vi "TickInd (SubVI).vi"(8 "error in (no error)":errorcluster, 11 "Tick":i32) -> (0 "error out":errorcluster)   [LabVIEW 2017]
uses:
  Global_SNK3_HF.vi
panel:
  out "subarray 2":sgl[](array[numeric])
  out "subarray":sgl[](array[numeric])
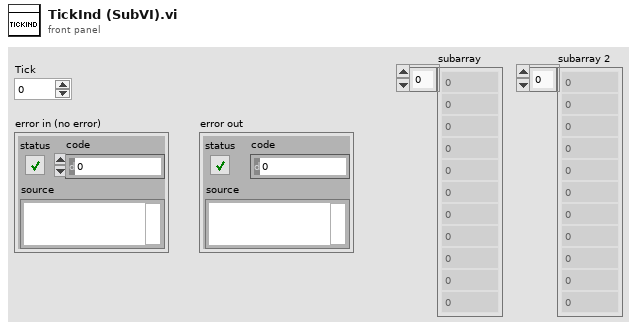
[diagram p1: front panel]
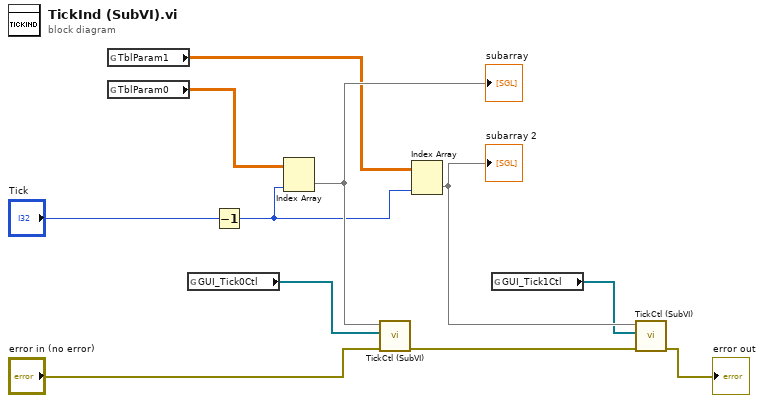
[diagram p0: block diagram]
diagram:
  n1 = global read "Global_SNK3_HF.vi" "TblParam1"() -> (w1:sgl[][])
  n2 = global read "Global_SNK3_HF.vi" "TblParam0"() -> (w2:sgl[][])
  n3 = global read "Global_SNK3_HF.vi" "GUI_Tick0Ctl"() -> (w6:refnum<vi>[])
  n4 = Decrement(x="Tick") -> (x-1=w3:i32)
  n5 = Index Array(array=w2, index (col)=w3) -> (element=w5:sgl[])  [unwired: 1 in]
  "subarray" <- w5
  n6 = call "TickCtl (SubVI).vi"("error in (no error)"="error in (no error)", "GUI_TickCtl"=w6, "TblParam"=w5) -> ("error out"=w8:errorcluster)  [unwired: 8 in]
  n7 = Index Array(array=w1, index (col)=w3) -> (element=w10:sgl[])  [unwired: 1 in]
  "subarray 2" <- w10
  n8 = global read "Global_SNK3_HF.vi" "GUI_Tick1Ctl"() -> (w9:refnum<vi>[])
  n9 = call "TickCtl (SubVI).vi"("error in (no error)"=w8, "GUI_TickCtl"=w9, "TblParam"=w10) -> ("error out"=→"error out":errorcluster)  [unwired: 8 in]
